vi "Config Aout Limit Error.vi"(8 "error in":errorcluster, 9 "Loss (off)":enum16{"off", "on"}(ring), 10 "Capacitance (off)":enum16{"off", "on"}(ring), 11 "VISA resource name":refnum<visa-resource-name>) -> (0 "error out":errorcluster, 3 "VISA resource name out":refnum<visa-resource-name>)   [LabVIEW 2019, in "Andeen-Hagerling 2700(400 firmware).lvlib"]
doc: "Determine whether voltages that exceed either of the two ALimC or either of the two ALimL values will report an error or not."
uses:
  Andeen-Hagerling 2700(400 firmware).lvlib
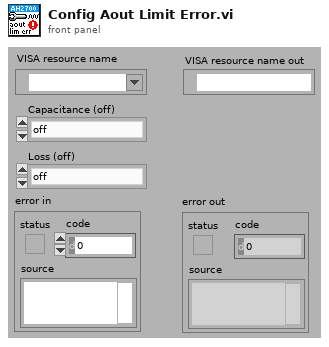
[diagram p1: front panel]
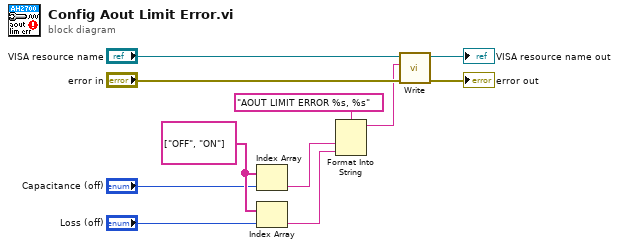
[diagram p0: block diagram]
diagram:
  w5 = string[] ["OFF", "ON"]
  n1 = Index Array(array=w5, index="Capacitance (off)") -> (element=w2:string)
  n2 = Index Array(array=w5, index="Loss (off)") -> (element=w1:string)
  n3 = Format Into String(format string="AOUT LIMIT ERROR %s, %s", w2, w1) -> (resulting string=w6:string)  [unwired: 2 in, 1 out]
  n4 = call "Write.vi"("error in"="error in", "command"=w6, "VISA resource name"="VISA resource name") -> ("error out"=→"error out":errorcluster, "VISA resource name out"=→"VISA resource name out":refnum<visa-resource-name>)  [unwired: 7 in]
